vi "Blackman-Harris Window.vi"   [LabVIEW 2014, in "NI_AALPro.lvlib"]
doc: "Applies a three-term, Blackman-Harris window to the input signal <B>X</B>. Wire data to the <B>X</B> input to determine the polymorphic instance to use or manually select the instance."
uses:
  NI_AALPro.lvlib
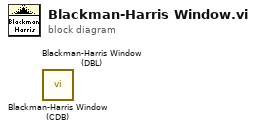
[diagram p0: block diagram]
diagram:
  n1 = call "Blackman-Harris Window (CDB).vi"() -> ()  [unwired: 1 in, 2 out]
  n2 = call "Blackman-Harris Window (DBL).vi"() -> ()  [unwired: 1 in, 2 out]
